vi "Play Sound.vi"(8 "error in (no error)":errorcluster, 11 "Sound LUMP IN":u8[](array[numeric])=[0, 0, 51, 0, 11, 5, 11, 5, 11, 6, 12, 9, 15, 10, 16, 13, 17, 14, 18, 18, 20, 20, 22, 22, 25, 24, 27, 24, 31, 21, 32, 19, 35, 18, 37, 16, 38, 14, 42, 13, 43, 11, 44, 10, 46, 8, 47, 8, 48, 5, 49, 3, 50, 0, 51]) -> (0 "error out":errorcluster)   [LabVIEW 2017]
uses:
  SoundFrequenciesList.ctl
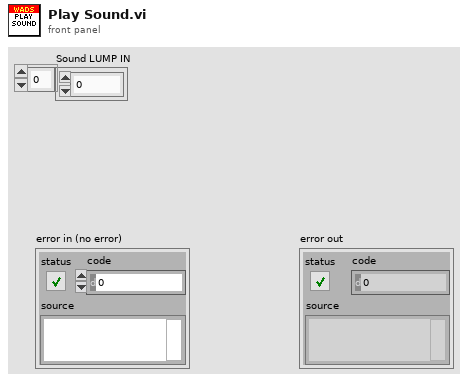
[diagram p1: front panel]
types:
  T1 = typedef "SoundFrequenciesList.ctl" = dbl[][]
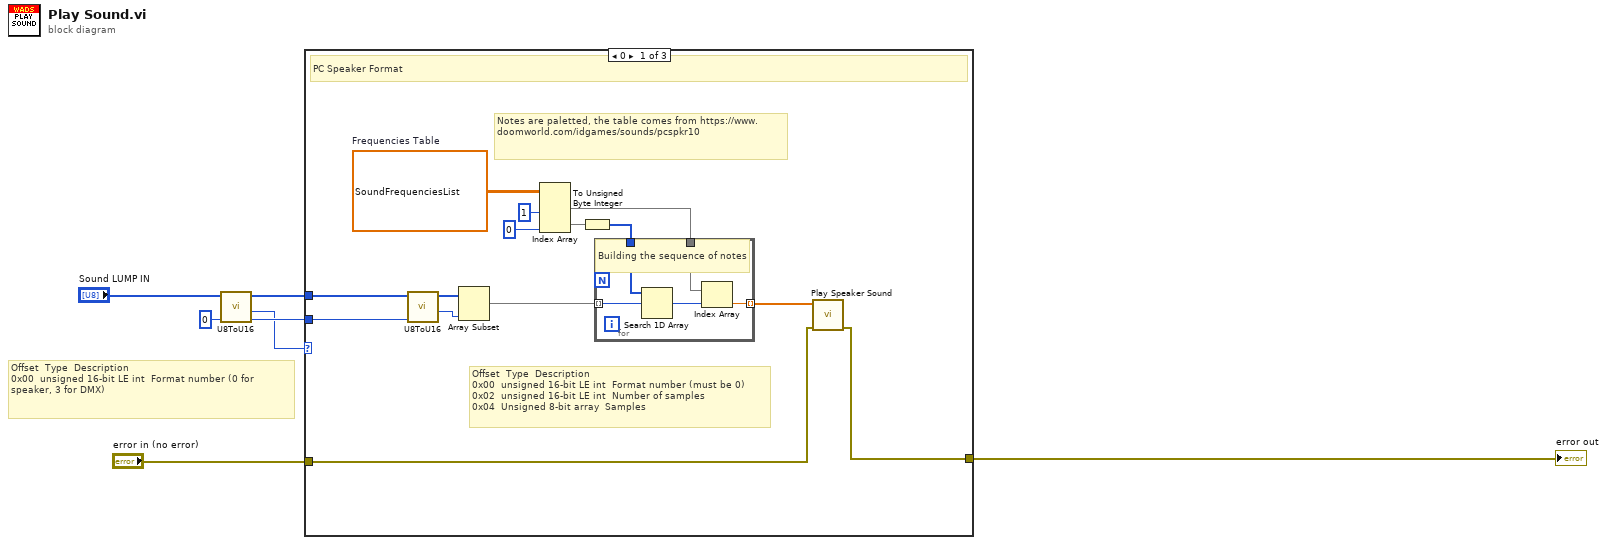
[diagram p0: block diagram]
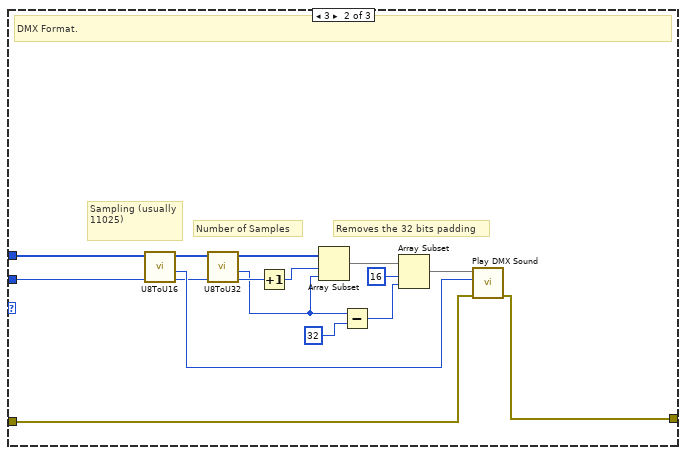
[diagram p2: hidden frame]
diagram:
  # "Offset \tType \tDescription\n0x00 \tunsigned 16-bit LE int \tFormat number (0 for speaker, 3 for DMX)"
  n1 = call "U8ToU16.vi"("Index"=u32 0, "Input U8 Array"="Sound LUMP IN") -> ("Index+2"=w3:u32, "Output U16"=w1:u16, "Output U8 Array"=w2:u8[])  [unwired: 3 in]
  n2 = case shown="0" w1 {
    tunnel: w2 -> [w11 w31 _]
    tunnel: w3 -> [w10 w30 _]
    tunnel: "error in (no error)" -> [w14 w40 w43]
    tunnel: [w13 w39 w43] -> w6
    frame 0 {
      w19 = T1 [[1.0, 175.0], [2.0, 180.02], [3.0, 185.01], [4.0, 190.02], [5.0, 196.02], [6.0, 202.02], [7.0, 208.01], [8.0, 214.02], [9.0, 220.02], [10.0, 226.02], [11.0, 233.04], [12.0, 240.02], [13.0, 247.03], [14.0, 254.03], [15.0, 262.0], [16.0, 269.03], [17.0, 277.03], [18.0, 285.04], [19.0, 294.03], [20.0, 302.07], [21.0, 311.04], [22.0, 320.05], [23.0, 330.06], [24.0, 339.06], [25.0, 349.08], [26.0, 359.06], [27.0, 370.09], [28.0, 381.08], [29.0, 392.1], [30.0, 403.1], [31.0, 415.01], [32.0, 427.05], [33.0, 440.12], [34.0, 453.16], [35.0, 466.08], [36.0, 480.15], [37.0, 494.07], [38.0, 508.16], [39.0, 523.09], [40.0, 539.16], [41.0, 554.19], [42.0, 571.17], [43.0, 587.19], [44.0, 604.14], [45.0, 622.09], [46.0, 640.11], [47.0, 659.21], [48.0, 679.1], [49.0, 698.17], [50.0, 719.21], [51.0, 740.18], [52.0, 762.41], [53.0, 784.47], [54.0, 807.29], [55.0, 831.48], [56.0, 855.32], [57.0, 880.57], [58.0, 906.67], [59.0, 932.17], [60.0, 960.69], [61.0, 988.55], [62.0, 1017.2], [63.0, 1046.64], [64.0, 1077.85], [65.0, 1109.93], [66.0, 1141.79], [67.0, 1175.54], [68.0, 1210.12], [69.0, 1244.19], [70.0, 1281.61], [71.0, 1318.43], [72.0, 1357.42], [73.0, 1397.16], [74.0, 1439.3], [75.0, 1480.37], [76.0, 1523.85], [77.0, 1569.97], [78.0, 1614.58], [79.0, 1661.81], [80.0, 1711.87], [81.0, 1762.45], [82.0, 1813.34], [83.0, 1864.34], [84.0, 1921.38], [85.0, 1975.46], [86.0, 2036.14], [87.0, 2093.29], [88.0, 2157.64], [89.0, 2217.8], [90.0, 2285.78], [91.0, 2353.41], [92.0, 2420.24], [93.0, 2490.98], [94.0, 2565.97], [95.0, 2639.77]]  # Frequencies Table
      # "Notes are paletted, the table comes from https://www.doomworld.com/idgames/sounds/pcspkr10"
      # "Offset \tType \tDescription\n0x00 \tunsigned 16-bit LE int \tFormat number (must be 0)\n0x02 \tunsigned 16-bit LE int \tNumber of samples\n0x04 \tUnsigned 8-bit array \tSamples"
      # "PC Speaker Format"
      n3 = call "U8ToU16.vi"("Index"=w10, "Input U8 Array"=w11) -> ("Output U16"=w8:u16, "Output U8 Array"=w9:u8[])  [unwired: 3 in, 1 out]
      n4 = Array Subset(array=w9, length=w8) -> (w12:u8[])  [unwired: 1 in]
      n5 = Index Array(array=w19, index (col) #1=1 ("disabled index (col)"), index (col) #2=0 ("disabled index (col)")) -> (element #1=w15:dbl[], element #2=w20:dbl[])  [unwired: 2 in]
      n6 = To Unsigned Byte Integer(number=w20) -> (unsigned 8bit integer=w16:u8[])
      n7 = for {
        tunnel: w16 -> [w26]
        tunnel: w15 -> [w25]
        tunnel: [w23] -> w21 mode=indexing
        tunnel: w12 -> [w22] mode=indexing
        # "Building the sequence of notes"
        n8 = Search 1D Array(1D array=w26, element=w22) -> (index of element=w24:i32)  [unwired: 1 in]
        n9 = Index Array(array=w25, index=w24) -> (element=w23:dbl)
      }
      n10 = call "Play Speaker Sound.vi"("error in (no error)"=w14, "Frequencies IN"=w21) -> ("error out"=w13:errorcluster)  [unwired: 9 in]
    }
    frame 3 {
      # "Number of Samples"
      # "Sampling (usually 11025)"
      # "Removes the 32 bits padding"
      # "DMX Format."
      n11 = call "U8ToU16.vi"("Index"=w30, "Input U8 Array"=w31) -> ("Index+2"=w27:u32, "Output U16"=w28:u16, "Output U8 Array"=w29:u8[])  [unwired: 3 in]
      n12 = call "U8ToU32.vi"("Index"=w27, "Input U8 Array"=w29) -> ("Index+4"=w41:u32, "Output U32"=w32:u32, "Output U8 Array"=w42:u8[])  [unwired: 3 in]
      n13 = Increment(x=w41) -> (x+1=w33:u32)
      n14 = Array Subset(array=w42, index=w33, length=w32) -> (w35:u8[])
      n15 = Subtract(x=w32, y=32 ("index")) -> (x-y=w37:u32)
      n16 = Array Subset(array=w35, index=16, length=w37) -> (w34:u8[])
      n17 = call "Play DMX Sound.vi"("error in (no error)"=w40, "Original Frq"=w28, "Frequencies IN"=w34) -> ("error out"=w39:errorcluster)  [unwired: 8 in]
    }
    frame Default {
      # "If a fancy sound format, do nothing..."
    }
  }
  "error out" <- w6
